vi "solar Menu (Initialize).vi"(6 "Is SOLAR UI? (F)":bool, 8 "error in (no error)":errorcluster, 10 "Targets":T1[](array[typedef]), 11 "MenuRef (NaN = All Menus)":refnum<k9>) -> (0 "error out":errorcluster)   [LabVIEW 2018]
doc: "This initializes the menu bar for each target."
uses:
  <vilib>/Utility/miscctls.llb/LVMenuShortCut.ctl
  solar_ctl Target Global.ctl
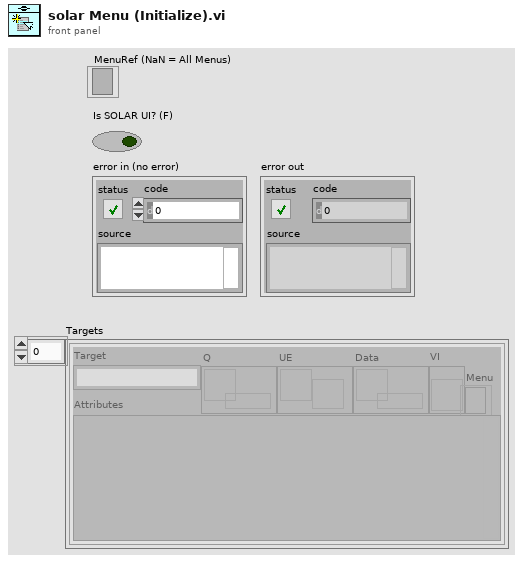
[diagram p1: front panel]
types:
  T1 = typedef "solar_ctl Target Global.ctl" = cluster{"Target":string, "Q":refnum<queue>, "UE":refnum<user-event>, "VI":refnum<vi>, "Menu":refnum<k9>, "Data":refnum<data-value>, "Attributes":variant}
  T2 = typedef "LVMenuShortCut.ctl" = cluster{"Include Shift Key?":bool, "Include Ctrl Key?":bool, "Shortcut Key":string}
  T3 = cluster{"Parent":string, "Items":cluster{"Label":string, "Tab":string, "Exe":bool, "Main":bool, "Disabled":bool, "Checked":bool, "Shortcut":T2}[]}[]
  T4 = enum32{"invalid app kind", "Development System", "Run Time System", "Student Edition", "Embedded LabVIEW", "Evaluation", "Custom"}
  T5 = cluster{"Label":string, "Tab":string, "Exe":bool, "Main":bool, "Disabled":bool, "Checked":bool, "Shortcut":T2}[]
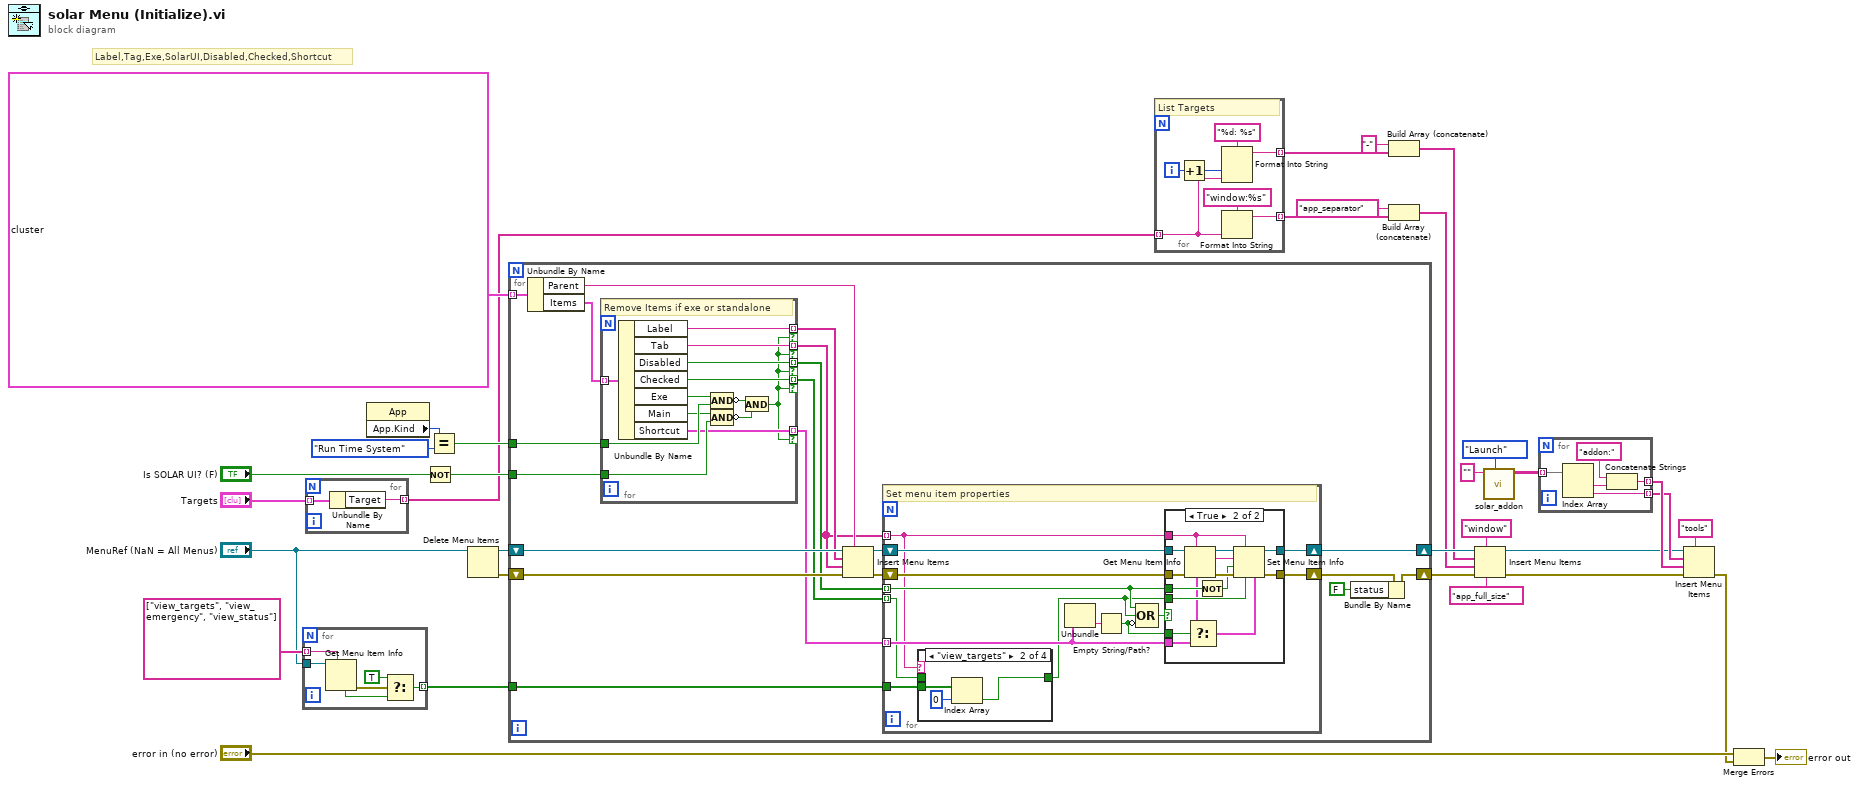
[diagram p0: block diagram]
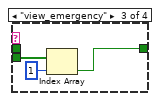
[diagram p3: hidden frame]
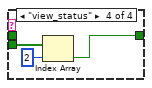
[diagram p4: hidden frame]
diagram:
  # "Label,Tag,Exe,SolarUI,Disabled,Checked,Shortcut"
  n1 = for {
    tunnel: "MenuRef (NaN = All Menus)" -> [w40]
    tunnel: string[] ["view_targets", "view_emergency", "view_status"] -> [w39] mode=indexing
    tunnel: [w36] -> w26 mode=indexing
    n2 = Get Menu Item Info(7:w39, 11:w40) -> (0:w38:errorcluster, 4:w37:bool)  [unwired: 1 in, 5 out]
    n3 = Select(t=TRUE, s=w38, f=w37) -> (s? t:f=w36:bool)
  }
  n4 = for {
    tunnel: [w42] -> w20 mode=indexing
    tunnel: "Targets" -> [w41] mode=indexing
    n5 = Unbundle By Name(w41) -> ("Target"=w42:string)
  }
  n6 = property class="App"() -> ("App.Kind"=w32:T4)  [unwired: 2 in, 2 out]
  n7 = Not(x="Is SOLAR UI? (F)") -> (.not. x?=w24:bool)
  n8 = Equal?(x=w32, y=T4."Run Time System") -> (x = y?=w29:bool)
  n9 = Delete Menu Items(9:"MenuRef (NaN = All Menus)") -> (0:w18:errorcluster, 3:w17:refnum<k9>)  [unwired: 3 in]
  n10 = for {
    shift-right: [w58] -> w12
    shift-left: w18 -> [w61]
    tunnel: T3 [{"Parent"="", "Items"=[{"Label"="File", "Tab"="file", "Exe"=FALSE, "Main"=FALSE, "Disabled"=FALSE, "Checked"=FALSE, "Shortcut"={"Include Shift Key?"=FALSE, "Include Ctrl Key?"=FALSE, "Shortcut Key"=""}}, {"Label"="Edit", "Tab"="edit", "Exe"=FALSE, "Main"=FALSE, "Disabled"=FALSE, "Checked"=FALSE, "Shortcut"={"Include Shift Key?"=FALSE, "Include Ctrl Key?"=FALSE, "Shortcut Key"=""}}, {"Label"="View", "Tab"="view", "Exe"=FALSE, "Main"=FALSE, "Disabled"=FALSE, "Checked"=FALSE, "Shortcut"={"Include Shift Key?"=FALSE, "Include Ctrl Key?"=FALSE, "Shortcut Key"=""}}, {"Label"="Tools", "Tab"="tools", "Exe"=FALSE, "Main"=FALSE, "Disabled"=FALSE, "Checked"=FALSE, "Shortcut"={"Include Shift Key?"=FALSE, "Include Ctrl Key?"=FALSE, "Shortcut Key"=""}}, {"Label"="Window", "Tab"="window", "Exe"=FALSE, "Main"=FALSE, "Disabled"=FALSE, "Checked"=FALSE, "Shortcut"={"Include Shift Key?"=FALSE, "Include Ctrl Key?"=FALSE, "Shortcut Key"=""}}, {"Label"="Help", "Tab"="help", "Exe"=FALSE, "Main"=FALSE, "Disabled"=FALSE, "Checked"=FALSE, "Shortcut"={"Include Shift Key?"=FALSE, "Include Ctrl Key?"=FALSE, "Shortcut Key"=""}}]}, {"Parent"="file", "Items"=[{"Label"="Explore...", "Tab"="file_explore", "Exe"=FALSE, "Main"=FALSE, "Disabled"=FALSE, "Checked"=FALSE, "Shortcut"={"Include Shift Key?"=FALSE, "Include Ctrl Key?"=FALSE, "Shortcut Key"=""}}, {"Label"="Export...", "Tab"="file_export", "Exe"=FALSE, "Main"=FALSE, "Disabled"=FALSE, "Checked"=FALSE, "Shortcut"={"Include Shift Key?"=FALSE, "Include Ctrl Key?"=FALSE, "Shortcut Key"=""}}, {"Label"="-", "Tab"="app_separator", "Exe"=FALSE, "Main"=FALSE, "Disabled"=FALSE, "Checked"=FALSE, "Shortcut"={"Include Shift Key?"=FALSE, "Include Ctrl Key?"=FALSE, "Shortcut Key"=""}}, {"Label"="Exit", "Tab"="app_close", "Exe"=FALSE, "Main"=FALSE, "Disabled"=FALSE, "Checked"=FALSE, "Shortcut"={"Include Shift Key?"=FALSE, "Include Ctrl Key?"=FALSE, "Shortcut Key"=""}}]}, {"Parent"="file_explore", "Items"=[{"Label"="App", "Tab"="file_explore_app", "Exe"=FALSE, "Main"=FALSE, "Disabled"=FALSE, "Checked"=FALSE, "Shortcut"={"Include Shift Key?"=FALSE, "Include Ctrl Key?"=FALSE, "Shortcut Key"=""}}, {"Label"="Configs", "Tab"="file_explore_configs", "Exe"=FALSE, "Main"=FALSE, "Disabled"=FALSE, "Checked"=FALSE, "Shortcut"={"Include Shift Key?"=FALSE, "Include Ctrl Key?"=FALSE, "Shortcut Key"=""}}, {"Label"="Cosmos", "Tab"="file_explore_cosmos", "Exe"=FALSE, "Main"=FALSE, "Disabled"=FALSE, "Checked"=FALSE, "Shortcut"={"Include Shift Key?"=FALSE, "Include Ctrl Key?"=FALSE, "Shortcut Key"=""}}, {"Label"="Logs", "Tab"="file_explore_logs", "Exe"=FALSE, "Main"=FALSE, "Disabled"=FALSE, "Checked"=FALSE, "Shortcut"={"Include Shift Key?"=FALSE, "Include Ctrl Key?"=FALSE, "Shortcut Key"=""}}]}, {"Parent"="file_export", "Items"=[{"Label"="Screenshots", "Tab"="file_export_screenshots", "Exe"=FALSE, "Main"=FALSE, "Disabled"=FALSE, "Checked"=FALSE, "Shortcut"={"Include Shift Key?"=FALSE, "Include Ctrl Key?"=FALSE, "Shortcut Key"=""}}, {"Label"="COSMOS", "Tab"="file_export_cosmos", "Exe"=FALSE, "Main"=FALSE, "Disabled"=FALSE, "Checked"=FALSE, "Shortcut"={"Include Shift Key?"=FALSE, "Include Ctrl Key?"=FALSE, "Shortcut Key"=""}}]}, {"Parent"="edit", "Items"=[{"Label"="Cut", "Tab"="app_cut", "Exe"=FALSE, "Main"=FALSE, "Disabled"=FALSE, "Checked"=FALSE, "Shortcut"={"Include Shift Key?"=FALSE, "Include Ctrl Key?"=FALSE, "Shortcut Key"=""}}, {"Label"="Copy", "Tab"="app_copy", "Exe"=FALSE, "Main"=FALSE, "Disabled"=FALSE, "Checked"=FALSE, "Shortcut"={"Include Shift Key?"=FALSE, "Include Ctrl Key?"=FALSE, "Shortcut Key"=""}}, {"Label"="Paste", "Tab"="app_paste", "Exe"=FALSE, "Main"=FALSE, "Disabled"=FALSE, "Checked"=FALSE, "Shortcut"={"Include Shift Key?"=FALSE, "Include Ctrl Key?"=FALSE, "Shortcut Key"=""}}, {"Label"="-", "Tab"="app_separator", "Exe"=TRUE, "Main"=FALSE, "Disabled"=FALSE, "Checked"=FALSE, "Shortcut"={"Include Shift Key?"=FALSE, "Include Ctrl Key?"=FALSE, "Shortcut Key"=""}}, {"Label"="Select All", "Tab"="app_select_all", "Exe"=TRUE, "Main"=FALSE, "Disabled"=FALSE, "Checked"=FALSE, "Shortcut"={"Include Shift Key?"=FALSE, "Include Ctrl Key?"=FALSE, "Shortcut Key"=""}}]}, {"Parent"="view", "Items"=[{"Label"="Targets", "Tab"="view_targets", "Exe"=FALSE, "Main"=TRUE, "Disabled"=FALSE, "Checked"=TRUE, "Shortcut"={"Include Shift Key?"=FALSE, "Include Ctrl Key?"=FALSE, "Shortcut Key"=""}}, {"Label"="Emergency Stop", "Tab"="view_emergency", "Exe"=FALSE, "Main"=TRUE, "Disabled"=FALSE, "Checked"=TRUE, "Shortcut"={"Include Shift Key?"=FALSE, "Include Ctrl Key?"=FALSE, "Shortcut Key"=""}}, {"Label"="Status", "Tab"="view_status", "Exe"=FALSE, "Main"=TRUE, "Disabled"=FALSE, "Checked"=TRUE, "Shortcut"={"Include Shift Key?"=FALSE, "Include Ctrl Key?"=FALSE, "Shortcut Key"=""}}, {"Label"="-", "Tab"="app_separator", "Exe"=FALSE, "Main"=TRUE, "Disabled"=FALSE, "Checked"=FALSE, "Shortcut"={"Include Shift Key?"=FALSE, "Include Ctrl Key?"=FALSE, "Shortcut Key"=""}}, {"Label"="Show All", "Tab"="view_show_all", "Exe"=FALSE, "Main"=TRUE, "Disabled"=FALSE, "Checked"=FALSE, "Shortcut"={"Include Shift Key?"=FALSE, "Include Ctrl Key?"=FALSE, "Shortcut Key"=""}}, {"Label"="Hide All", "Tab"="view_hide_all", "Exe"=FALSE, "Main"=TRUE, "Disabled"=FALSE, "Checked"=FALSE, "Shortcut"={"Include Shift Key?"=FALSE, "Include Ctrl Key?"=FALSE, "Shortcut Key"=""}}, {"Label"="-", "Tab"="app_separator", "Exe"=FALSE, "Main"=TRUE, "Disabled"=FALSE, "Checked"=FALSE, "Shortcut"={"Include Shift Key?"=FALSE, "Include Ctrl Key?"=FALSE, "Shortcut Key"=""}}, {"Label"="Refresh", "Tab"="view_refresh", "Exe"=FALSE, "Main"=FALSE, "Disabled"=FALSE, "Checked"=FALSE, "Shortcut"={"Include Shift Key?"=FALSE, "Include Ctrl Key?"=FALSE, "Shortcut Key"="F5"}}]}, {"Parent"="tools", "Items"=[{"Label"="New SOLAR Addon...", "Tab"="tools_new_addon", "Exe"=FALSE, "Main"=FALSE, "Disabled"=FALSE, "Checked"=FALSE, "Shortcut"={"Include Shift Key?"=FALSE, "Include Ctrl Key?"=FALSE, "Shortcut Key"=""}}, {"Label"="-", "Tab"="app_separator", "Exe"=FALSE, "Main"=FALSE, "Disabled"=FALSE, "Checked"=FALSE, "Shortcut"={"Include Shift Key?"=FALSE, "Include Ctrl Key?"=FALSE, "Shortcut Key"=""}}]}, {"Parent"="window", "Items"=[{"Label"="Show Panel or Diagram", "Tab"="app_show_panel_diagram", "Exe"=TRUE, "Main"=FALSE, "Disabled"=FALSE, "Checked"=FALSE, "Shortcut"={"Include Shift Key?"=FALSE, "Include Ctrl Key?"=FALSE, "Shortcut Key"=""}}, {"Label"="-", "Tab"="app_separator", "Exe"=TRUE, "Main"=FALSE, "Disabled"=FALSE, "Checked"=FALSE, "Shortcut"={"Include Shift Key?"=FALSE, "Include Ctrl Key?"=FALSE, "Shortcut Key"=""}}, {"Label"="Position", "Tab"="window_position", "Exe"=FALSE, "Main"=FALSE, "Disabled"=FALSE, "Checked"=FALSE, "Shortcut"={"Include Shift Key?"=FALSE, "Include Ctrl Key?"=FALSE, "Shortcut Key"=""}}, {"Label"="-", "Tab"="app_separator", "Exe"=FALSE, "Main"=FALSE, "Disabled"=FALSE, "Checked"=FALSE, "Shortcut"={"Include Shift Key?"=FALSE, "Include Ctrl Key?"=FALSE, "Shortcut Key"=""}}, {"Label"="Full Size", "Tab"="app_full_size", "Exe"=FALSE, "Main"=FALSE, "Disabled"=FALSE, "Checked"=FALSE, "Shortcut"={"Include Shift Key?"=FALSE, "Include Ctrl Key?"=FALSE, "Shortcut Key"=""}}, {"Label"="-", "Tab"="app_separator", "Exe"=FALSE, "Main"=FALSE, "Disabled"=FALSE, "Checked"=FALSE, "Shortcut"={"Include Shift Key?"=FALSE, "Include Ctrl Key?"=FALSE, "Shortcut Key"=""}}, {"Label"="Reload", "Tab"="window_reload", "Exe"=FALSE, "Main"=FALSE, "Disabled"=FALSE, "Checked"=FALSE, "Shortcut"={"Include Shift Key?"=FALSE, "Include Ctrl Key?"=FALSE, "Shortcut Key"=""}}]}, {"Parent"="window_position", "Items"=[{"Label"="Set", "Tab"="window_set_position", "Exe"=FALSE, "Main"=FALSE, "Disabled"=FALSE, "Checked"=FALSE, "Shortcut"={"Include Shift Key?"=FALSE, "Include Ctrl Key?"=FALSE, "Shortcut Key"=""}}, {"Label"="Reset", "Tab"="window_reset_position", "Exe"=FALSE, "Main"=FALSE, "Disabled"=FALSE, "Checked"=FALSE, "Shortcut"={"Include Shift Key?"=FALSE, "Include Ctrl Key?"=FALSE, "Shortcut Key"=""}}, {"Label"="-", "Tab"="app_separator", "Exe"=FALSE, "Main"=FALSE, "Disabled"=FALSE, "Checked"=FALSE, "Shortcut"={"Include Shift Key?"=FALSE, "Include Ctrl Key?"=FALSE, "Shortcut Key"=""}}, {"Label"="Clear", "Tab"="window_clear_position", "Exe"=FALSE, "Main"=FALSE, "Disabled"=FALSE, "Checked"=FALSE, "Shortcut"={"Include Shift Key?"=FALSE, "Include Ctrl Key?"=FALSE, "Shortcut Key"=""}}]}, {"Parent"="help", "Items"=[{"Label"="Show Context", "Tab"="app_show_help", "Exe"=FALSE, "Main"=FALSE, "Disabled"=FALSE, "Checked"=FALSE, "Shortcut"={"Include Shift Key?"=FALSE, "Include Ctrl Key?"=FALSE, "Shortcut Key"=""}}, {"Label"="-", "Tab"="app_separator", "Exe"=TRUE, "Main"=FALSE, "Disabled"=FALSE, "Checked"=FALSE, "Shortcut"={"Include Shift Key?"=FALSE, "Include Ctrl Key?"=FALSE, "Shortcut Key"=""}}, {"Label"="SOLAR Help...", "Tab"="help_solar", "Exe"=TRUE, "Main"=FALSE, "Disabled"=FALSE, "Checked"=FALSE, "Shortcut"={"Include Shift Key?"=FALSE, "Include Ctrl Key?"=FALSE, "Shortcut Key"=""}}, {"Label"="-", "Tab"="app_separator", "Exe"=FALSE, "Main"=FALSE, "Disabled"=FALSE, "Checked"=FALSE, "Shortcut"={"Include Shift Key?"=FALSE, "Include Ctrl Key?"=FALSE, "Shortcut Key"=""}}, {"Label"="About SOLAR...", "Tab"="help_about", "Exe"=FALSE, "Main"=FALSE, "Disabled"=FALSE, "Checked"=FALSE, "Shortcut"={"Include Shift Key?"=FALSE, "Include Ctrl Key?"=FALSE, "Shortcut Key"=""}}]}] -> [w57] mode=indexing
    shift-right: [w49] -> w16
    shift-left: w17 -> [w60]
    tunnel: w29 -> [w48]
    tunnel: w24 -> [w47]
    tunnel: w26 -> [w43]
    n11 = Unbundle By Name(w57) -> ("Parent"=w56:string, "Items"=w55:T5)
    n12 = for {
      tunnel: w55 -> [w114] mode=indexing
      tunnel: [w113] -> w54 mode=indexing if=w102
      tunnel: [w112] -> w50 mode=indexing if=w102
      tunnel: w48 -> [w110]
      tunnel: w47 -> [w106]
      tunnel: [w105] -> w46 mode=indexing if=w102
      tunnel: [w104] -> w45 mode=indexing if=w102
      tunnel: [w103] -> w44 mode=indexing if=w102
      # "Remove Items if exe or standalone"
      n13 = Unbundle By Name(w114) -> ("Label"=w113:string, "Tab"=w112:string, "Disabled"=w105:bool, "Checked"=w104:bool, "Exe"=w111:bool, "Main"=w109:bool, "Shortcut"=w103:T2)
      n14 = Compound Arithmetic op=AND(w111, w110) -> (invert w108:bool)
      n15 = Compound Arithmetic op=AND(w109, w106) -> (invert w107:bool)
      n16 = And(x=w108, y=w107) -> (x .and. y?=w102:bool)
    }
    n17 = Insert Menu Items(5:w56, 6:w61, 7:w50, 8:w54, 9:w60) -> (0:w52:errorcluster, 3:w53:refnum<k9>)  [unwired: 1 in, 1 out]
    n18 = for {
      shift-right: [w72] -> w51
      shift-left: w52 -> [w73]
      tunnel: w50 -> [w65] mode=indexing
      shift-right: [w71] -> w49
      shift-left: w53 -> [w74]
      tunnel: w46 -> [w69] mode=indexing
      tunnel: w45 -> [w63] mode=indexing
      tunnel: w44 -> [w68] mode=indexing
      tunnel: w43 -> [w64]
      # "Set menu item properties"
      n19 = case shown="\"view_targets\"" w65 {
        tunnel: w64 -> [_ w78 w81 w84]
        tunnel: [w75 w77 w80 w83] -> w62
        tunnel: w63 -> [w75 _ _ _]
        frame Default {
        }
        frame "view_targets" {
          n20 = Index Array(array=w78, index=0) -> (element=w77:bool)
        }
        frame "view_emergency" {
          n21 = Index Array(array=w81, index=1) -> (element=w80:bool)
        }
        frame "view_status" {
          n22 = Index Array(array=w84, index=2) -> (element=w83:bool)
        }
      }
      n23 = Unbundle(w68) -> ("Shortcut Key"=w67:string)  [unwired: 2 out]
      n24 = Empty String/Path?(string/path=w67) -> (empty?=w66:bool)
      n25 = Compound Arithmetic op=OR(w69, w62, invert w66) -> (w70:bool)
      n26 = case shown="True" w70 {
        tunnel: w74 -> [w86 w98]
        tunnel: w73 -> [w85 w97]
        tunnel: [w85 w96] -> w72
        tunnel: w65 -> [_ w95]
        tunnel: [w86 w94] -> w71
        tunnel: w69 -> [_ w93]
        tunnel: w62 -> [_ w92]
        tunnel: w68 -> [_ w88]
        tunnel: w66 -> [_ w87]
        frame False {
        }
        frame True {
          n27 = Get Menu Item Info(7:w95, 8:w97, 11:w98) -> (0:w99:errorcluster, 2:w101:string, 3:w100:refnum<k9>, 6:w89:T2)  [unwired: 3 out]
          n28 = Select(t=w89, s=w87, f=w88) -> (s? t:f=w90:T2)
          n29 = Not(x=w93) -> (.not. x?=w91:bool)
          n30 = Set Menu Item Info(4:w90, 6:w92, 7:w95, 8:w99, 9:w91, 10:w101, 11:w100) -> (0:w96:errorcluster, 3:w94:refnum<k9>)
        }
      }
    }
    n31 = Bundle By Name(cluster=w51, "status"=FALSE) -> (w58:errorcluster)
  }
  n32 = for {
    tunnel: w20 -> [w115] mode=indexing
    tunnel: [w117] -> w14 mode=indexing
    tunnel: [w116] -> w13 mode=indexing
    i -> [w121]
    # "List Targets"
    n33 = Increment(x=w121) -> (x+1=w120:i32)
    n34 = Format Into String(format string="%d: %s", w120, w115) -> (resulting string=w117:string)  [unwired: 2 in, 1 out]
    n35 = Format Into String(format string="window:%s", w115) -> (resulting string=w116:string)  [unwired: 2 in, 1 out]
  }
  n36 = Build Array (concatenate)("-", w14) -> (w10:string[])
  n37 = Build Array (concatenate)("app_separator", w13) -> (w11:string[])
  n38 = Insert Menu Items(4:"app_full_size" ("after item"), 5:"window" ("menu tag"), 6:w12, 7:w11, 8:w10, 9:w16) -> (0:w5:errorcluster, 3:w4:refnum<k9>)  [unwired: 1 out]
  n39 = call "solar_addon.vi"("Action (Launch)"=enum8{"Launch", "Initialize", "Shutdown"}."Launch", "Launch Addon VI"="") -> ("Addons (vi,title)"=w23:string[][])  [unwired: 8 in, 1 out]
  n40 = for {
    tunnel: w23 -> [w126] mode=indexing
    tunnel: [w123] -> w22 mode=indexing
    tunnel: [w122] -> w21 mode=indexing
    n41 = Index Array(array=w126) -> (element #1=w125:string, element #2=w122:string)  [unwired: 2 in]
    n42 = Concatenate Strings("addon:", w125) -> (w123:string)
  }
  n43 = Insert Menu Items(5:"tools" ("menu tag"), 6:w5, 7:w22, 8:w21, 9:w4) -> (0:w28:errorcluster)  [unwired: 1 in, 2 out]
  n44 = Merge Errors("error in (no error)", w28) -> (→"error out":errorcluster)
